vi "find-path.vi"(4 "Start Y":i32, 6 "Start X":i32, 7 "Obstacles":i32[][](array[numeric]), 9 "Numeric":dbl, 10 "Numeric 2":dbl, 11 "Destination":i32[](array[numeric])) -> (2 "Instructions":i32[][](array[numeric]), 3 "appended array":dbl[][](array[numeric]))   [LabVIEW 2015]
uses:
  <vilib>/robotics/Navigation/shared/WorldMap/OccupancyGridWorldMap/NI_Robotics_OccupancyGridWorldMap.lvclass
  <vilib>/robotics/Navigation/NI_Robotics_Navigation .lvlib
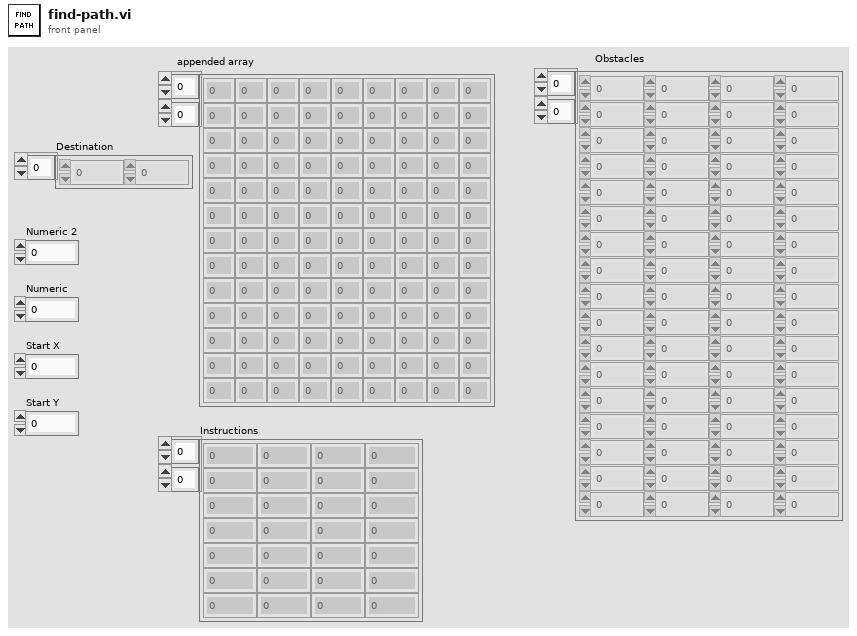
[diagram p1: front panel]
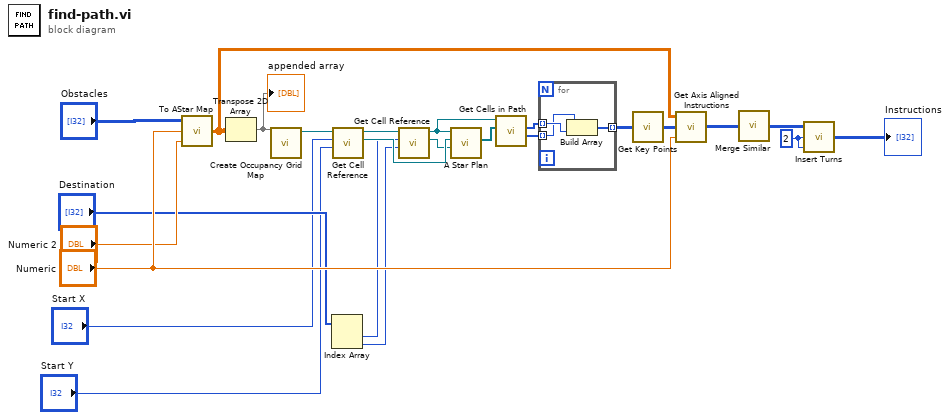
[diagram p0: block diagram]
diagram:
  w18 = 2 ("Forward Turn Movement")
  n1 = call "To AStar Map.vi"("empty value"="Numeric 2", "Wall value"="Numeric", "Obstacles"="Obstacles") -> ("a star map"=w1:dbl[][])
  n2 = Transpose 2D Array(2D array=w1) -> (transposed array=w2:dbl[][])
  "appended array" <- w2
  n3 = call <vilib>:"Create Occupancy Grid Map.vi"("occupancy grid"=w2) -> ("map reference out"=w3:refnum<data-value>)  [unwired: 9 in, 1 out]
  n4 = Index Array(array="Destination") -> (element #1=w8:i32, element #2=w9:i32)  [unwired: 2 in]
  n5 = call <vilib>:"Get Cell Reference.vi"("y"="Start Y", "x"="Start X", "map reference in"=w3) -> ("cell reference"=w11:refnum<data-value>, "map reference out"=w6:refnum<data-value>)  [unwired: 5 in, 2 out]
  n6 = call <vilib>:"Get Cell Reference.vi"("y"=w9, "x"=w8, "map reference in"=w6) -> ("cell reference"=w10:refnum<data-value>, "map reference out"=w13:refnum<data-value>)  [unwired: 5 in, 2 out]
  n7 = call <vilib>:"A Star Plan.vi"("goal reference"=w10, "start reference"=w11, "map reference in"=w13) -> ("path references"=w12:refnum<data-value>[])  [unwired: 5 in, 3 out]
  n8 = call <vilib>:"Get Cells in Path.vi"("path references"=w12, "map reference in"=w13) -> ("y coordinates"=w15:i32[], "x coordinates"=w14:i32[])  [unwired: 6 in, 2 out]
  n9 = for {
    tunnel: w14 -> [w26] mode=indexing
    tunnel: w15 -> [w25] mode=indexing
    tunnel: [w27] -> w16 mode=indexing
    n10 = Build Array(w25, w26) -> (w27:i32[])
  }
  n11 = call "Get Key Points.vi"("Path"=w16) -> ("Key Points"=w22:i32[][])
  n12 = call "Get Axis Aligned Instructions.vi"("Wall value"="Numeric", "Key Points"=w22, "obstacles"=w1) -> ("AA Instructions"=w24:i32[][])
  n13 = call "Merge Similar.vi"("AA Instructions"=w24) -> ("Merged Instructions"=w17:i32[][])
  n14 = call "Insert Turns.vi"("Sideways Turn Movement"=w18, "Forward Turn Movement"=w18, "Merged Instructions"=w17) -> ("Instructions"=→"Instructions":i32[][])
